vi "TempMonitor_SetLimits_ConfirmLimits.vi"(9 "Limit (C)":i32=-10, 10 "Which Limit?":enum16{"Low", "High"}(ring), 11 "Serial Port to Use":refnum<visa-resource-name>="COM8") -> (0 "Error Out":errorcluster, 2 "Response Message":string, 3 "Pass":bool)   [LabVIEW 2012]
doc: "Set the Temperature Limit for the DUT over UART. Then read back the limit over UART to confirm that it was accepted and stored by the DUT. Either a Low or High limit can be checked."
uses:
  TempMonitor_Command_Enumerations.vi
panel:
  out "Layer2 Payload 1":string
  out "A Packet Acked 1":bool
  out "Ack Received 1":bool
  out "Layer2 Payload 2":string
  out "A Packet Acked 2":bool
  out "Ack Received 2":bool
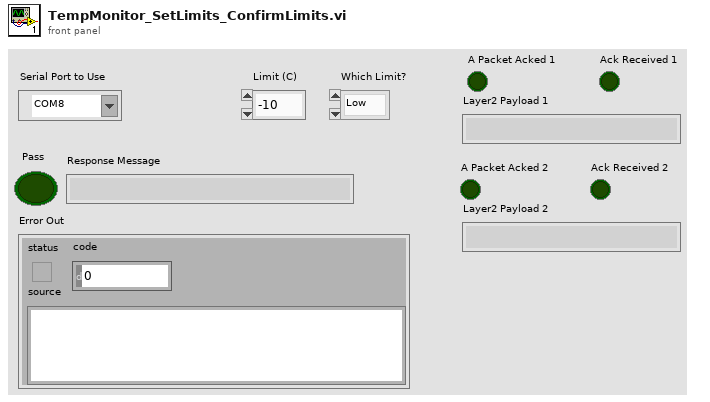
[diagram p1: front panel]
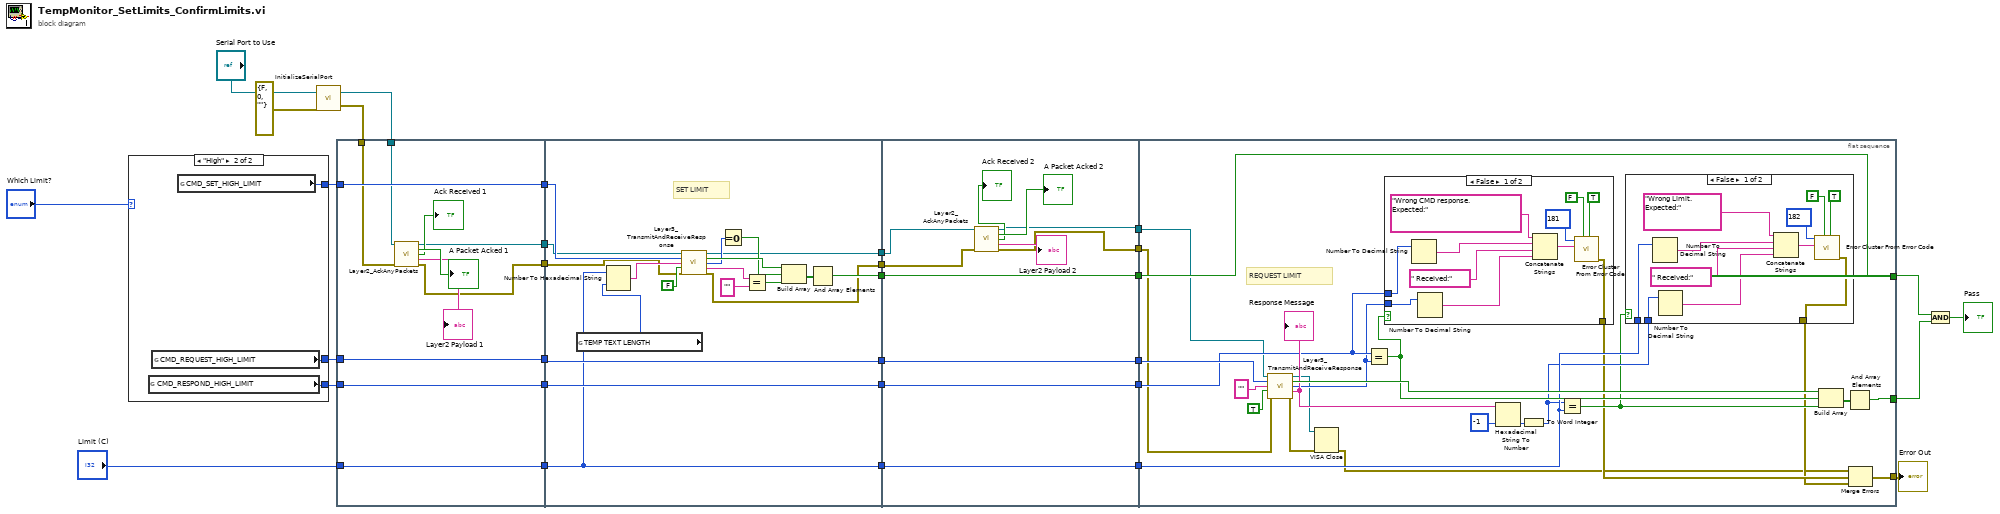
[diagram p0: block diagram]
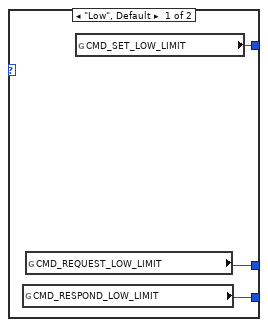
[diagram p2: hidden frame]
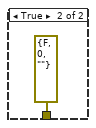
[diagram p3: hidden frame]
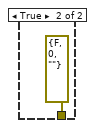
[diagram p4: hidden frame]
diagram:
  n1 = case shown="\"High\"" "Which Limit?" {
    tunnel: [w34 w37] -> w31
    tunnel: [w33 w36] -> w30
    tunnel: [w32 w35] -> w29
    frame "Low", Default {
      n2 = global read "TempMonitor_Command_Enumerations.vi" "CMD_RESPOND_LOW_LIMIT"() -> (w32:u16)
      n3 = global read "TempMonitor_Command_Enumerations.vi" "CMD_REQUEST_LOW_LIMIT"() -> (w33:u16)
      n4 = global read "TempMonitor_Command_Enumerations.vi" "CMD_SET_LOW_LIMIT"() -> (w34:u16)
    }
    frame "High" {
      n5 = global read "TempMonitor_Command_Enumerations.vi" "CMD_RESPOND_HIGH_LIMIT"() -> (w35:u16)
      n6 = global read "TempMonitor_Command_Enumerations.vi" "CMD_REQUEST_HIGH_LIMIT"() -> (w36:u16)
      n7 = global read "TempMonitor_Command_Enumerations.vi" "CMD_SET_HIGH_LIMIT"() -> (w37:u16)
    }
  }
  n8 = call "InitializeSerialPort.vi"("error in (no error)"=errorcluster {"status"=FALSE, "code"=0, "source"=""}, "Serial Port to Use"="Serial Port to Use") -> ("error out"=w8:errorcluster, "Configured Serial Port Identifier"=w7:refnum<visa-resource-name>)
  n9 = flat-sequence {
    tunnel: "Limit (C)" -> [w45]
    tunnel: w29 -> [w46]
    tunnel: w30 -> [w47]
    tunnel: w31 -> [w48]
    tunnel: [w48] -> w18
    tunnel: [w47] -> w17
    tunnel: [w46] -> w16
    tunnel: [w45] -> w15
    tunnel: w7 -> [w44]
    tunnel: w8 -> [w40]
    tunnel: [w39] -> w6
    tunnel: [w38] -> w5
    tunnel: [w60] -> w26
    tunnel: [w59] -> w24
    tunnel: [w57] -> w22
    tunnel: [w56] -> w20
    tunnel: w18 -> [w54]
    tunnel: w17 -> [w60]
    tunnel: w16 -> [w59]
    tunnel: w15 -> [w57]
    tunnel: w6 -> [w53]
    tunnel: w5 -> [w52]
    tunnel: [w51] -> w4
    tunnel: [w50] -> w3
    tunnel: w26 -> [w78]
    tunnel: [w78] -> w25
    tunnel: w24 -> [w77]
    tunnel: [w77] -> w23
    tunnel: w22 -> [w76]
    tunnel: [w76] -> w21
    tunnel: w20 -> [w75]
    tunnel: [w75] -> w19
    tunnel: w4 -> [w71]
    tunnel: w3 -> [w70]
    tunnel: [w69] -> w2
    tunnel: [w68] -> w1
    tunnel: w25 -> [w98]
    tunnel: w23 -> [w92]
    tunnel: w21 -> [w88]
    tunnel: [w90] -> w10
    tunnel: w19 -> [w90]
    tunnel: [w95] -> w11
    tunnel: [w93] -> w13
    tunnel: w2 -> [w79]
    tunnel: w1 -> [w80]
    frame #0 {
      n10 = call "Layer2_AckAnyPackets.vi"("Serial Port to Use"=w44, "Error In"=w40) -> ("Serial Port to Use (out)"=w39:refnum<visa-resource-name>, "A Packet Acked"=→"A Packet Acked 1":bool, "Ack Received"=→"Ack Received 1":bool, "Layer2 Payload"=→"Layer2 Payload 1":string, "Error Out"=w38:errorcluster)  [unwired: 9 in]
    }
    frame #1 {
      # "SET LIMIT"
      n11 = global read "TempMonitor_Command_Enumerations.vi" "TEMP TEXT LENGTH"() -> (w49:u8)
      n12 = Number To Hexadecimal String(1:w49, 2:w57) -> (0:w58:string)
      n13 = call "Layer3_TransmitAndReceiveResponse.vi"("Serial Port to Use"=w53, "CMD"=w54, "Message"=w58, "Expecting Response"=FALSE, "error in (no error)"=w52) -> ("Serial Port to Use (out)"=w51:refnum<visa-resource-name>, "Success"=w62:bool, "Response CMD"=w55:u16, "Response Message"=w64:string, "Error Out"=w50:errorcluster)  [unwired: 6 in]
      n14 = Equal To 0?(x=w55) -> (x = 0?=w61:bool)
      n15 = Equal?(x=w64, y="" ("x")) -> (x = y?=w63:bool)
      n16 = Build Array(w62, w61, w63) -> (w67:bool[])
      n17 = And Array Elements(Boolean array=w67) -> (logical AND=w56:bool)
    }
    frame #2 {
      n18 = call "Layer2_AckAnyPackets.vi"("Serial Port to Use"=w71, "Error In"=w70) -> ("Serial Port to Use (out)"=w68:refnum<visa-resource-name>, "A Packet Acked"=→"A Packet Acked 2":bool, "Ack Received"=→"Ack Received 2":bool, "Layer2 Payload"=→"Layer2 Payload 2":string, "Error Out"=w69:errorcluster)  [unwired: 9 in]
    }
    frame #3 {
      # "REQUEST LIMIT"
      n19 = call "Layer3_TransmitAndReceiveResponse.vi"("Serial Port to Use"=w80, "CMD"=w98, "Message"="", "Expecting Response"=TRUE, "error in (no error)"=w79) -> ("Serial Port to Use (out)"=w81:refnum<visa-resource-name>, "Success"=w99:bool, "Response CMD"=w91:u16, "Response Message"=w97:string, "Error Out"=w83:errorcluster)  [unwired: 6 in]
      "Response Message" <- w97
      n20 = VISA Close(VISA resource name=w81, error in (no error)=w83) -> (error out=w82:errorcluster)
      n21 = Equal?(x=w92, y=w91) -> (x = y?=w89:bool)
      n22 = case shown="False" w89 {
        tunnel: w92 -> [w125 _]
        tunnel: w91 -> [w124 _]
        tunnel: [w115 errorcluster {"status"=FALSE, "code"=0, "source"=""} ("error out")] -> w85
        frame False {
          n23 = Number To Decimal String(number=w125) -> (decimal integer string=w122:string)  [unwired: 1 in]
          n24 = Number To Decimal String(number=w124) -> (decimal integer string=w121:string)  [unwired: 1 in]
          n25 = Concatenate Strings("Wrong CMD response. Expected:" ("error message (\"\")"), w122, " Received:" ("error message (\"\")"), w121) -> (w119:string)
          n26 = call <vilib>:"Error Cluster From Error Code.vi"("is warning? (False)"=TRUE, "show call chain? (False)"=FALSE, "error message (\"\")"=w119, "error code (0)"=181) -> ("error out"=w115:errorcluster)  [unwired: 5 in]
        }
        frame True {
        }
      }
      n27 = Hexadecimal String To Number(string=w97, default (0uL)=-1 ("default (0 U32)")) -> (number=w94:i32)  [unwired: 1 in, 1 out]
      n28 = To Word Integer(number=w94) -> (16bit integer=w87:i16)
      n29 = Equal?(x=w87, y=w88) -> (x = y?=w86:bool)
      n30 = case shown="False" w86 {
        tunnel: w88 -> [w105 _]
        tunnel: w87 -> [w104 _]
        tunnel: [w103 errorcluster {"status"=FALSE, "code"=0, "source"=""} ("error out")] -> w84
        frame False {
          n31 = Number To Decimal String(number=w105) -> (decimal integer string=w112:string)  [unwired: 1 in]
          n32 = Number To Decimal String(number=w104) -> (decimal integer string=w111:string)  [unwired: 1 in]
          n33 = Concatenate Strings("Wrong Limit. Expected:" ("error message (\"\")"), w112, " Received:" ("error message (\"\")"), w111) -> (w109:string)
          n34 = call <vilib>:"Error Cluster From Error Code.vi"("is warning? (False)"=TRUE, "show call chain? (False)"=FALSE, "error message (\"\")"=w109, "error code (0)"=182) -> ("error out"=w103:errorcluster)  [unwired: 5 in]
        }
        frame True {
        }
      }
      n35 = Build Array(w99, w89, w86) -> (w102:bool[])
      n36 = And Array Elements(Boolean array=w102) -> (logical AND=w95:bool)
      n37 = Merge Errors(w82, w85, w84) -> (w93:errorcluster)
    }
  }
  n38 = And(x=w10, y=w11) -> (x .and. y?=→"Pass":bool)
  "Error Out" <- w13
